vi "Update Command Settings.vi"(8 "error in (no error)":errorcluster, 10 "Command Settings":refnum<class "CommandSetting.lvclass">[](array[class]), 11 "WriteCommand in":refnum<class "WriteCommand.lvclass">) -> (0 "error out":errorcluster, 1 "Updated Count":u32, 2 "Added Count":u32, 3 "WriteCommand out":refnum<class "WriteCommand.lvclass">)   [LabVIEW 2023, in "HAF.lvlib" / "WriteCommand.lvclass"]
doc: "Adds to or updates existing Command Settings on the Command. Returns the number added and updated."
uses:
  WriteCommand.lvclass
  CommandSetting/CommandSetting.lvclass
  WriteCommand.lvclass/WriteCommand.ctl
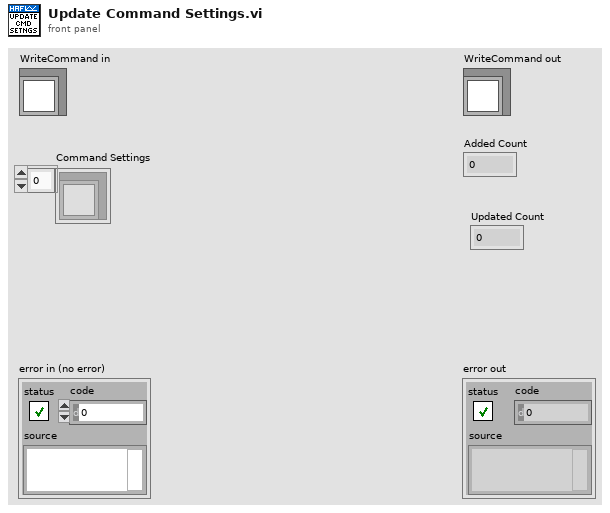
[diagram p1: front panel]
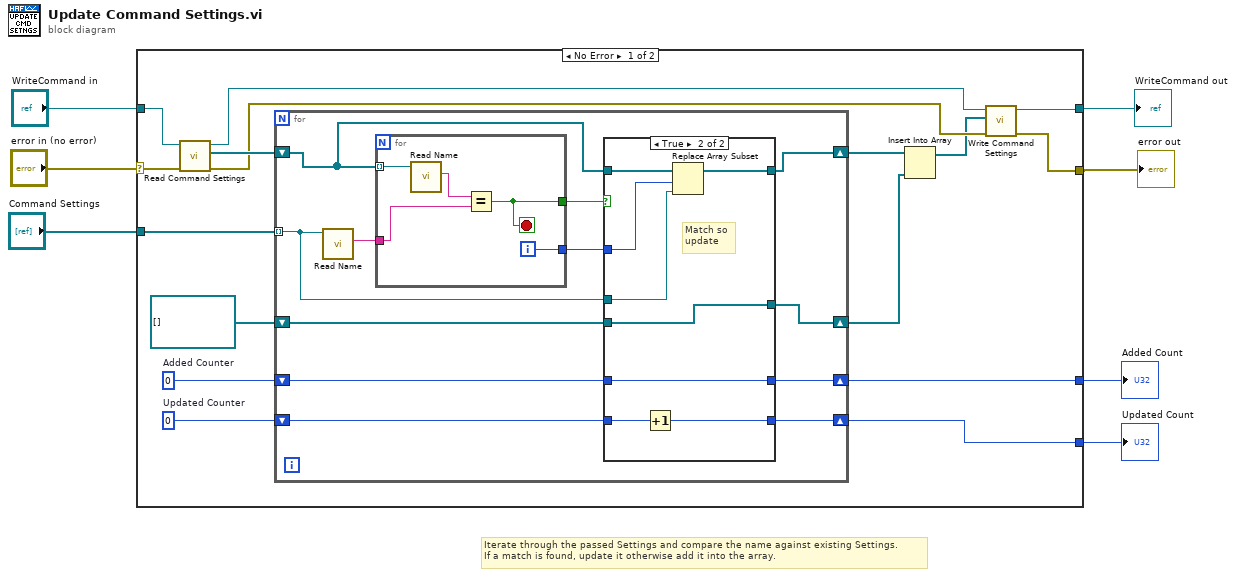
[diagram p0: block diagram]
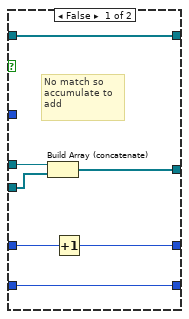
[diagram p2: hidden frame]
diagram:
  # "Iterate through the passed Settings and compare the name against existing Settings.\nIf a match is found, update it otherwise add it into the array."
  n1 = case shown="No Error" "error in (no error)" {
    selector: "error in (no error)" -> [w22 w57]
    tunnel: [w10 w57] -> w3
    tunnel: [w11 w56] -> w4
    tunnel: "WriteCommand in" -> [w23 w56]
    tunnel: "Command Settings" -> [w21 _]
    tunnel: [w9 _] -> w2
    tunnel: [w8 _] -> w1
    frame No Error {
      w18 = u32 0  # Updated Counter
      w19 = u32 0  # Added Counter
      n2 = call-dynamic "Read Command Settings.vi"("error in (no error)"=w22, "WriteCommand in"=w23) -> ("error out"=w14:errorcluster, "Command Settings"=w17:refnum<class "CommandSetting.lvclass">[], "WriteCommand out"=w13:refnum<class "WriteCommand.lvclass">)  [unwired: 7 in]
      n3 = for {
        tunnel: w21 -> [w32] mode=indexing
        shift-right: [w27] -> w15
        shift-left: refnum<class "CommandSetting.lvclass">[] [] -> [w31]
        shift-right: [w26] -> w9
        shift-left: w19 -> [w30]
        shift-right: [w25] -> w8
        shift-left: w18 -> [w29]
        shift-right: [w24] -> w16
        shift-left: w17 -> [w28]
        n4 = call-dynamic "Read Name.vi"("Setting in"=w32) -> ("Name"=w35:string)  [unwired: 8 in, 2 out]
        n5 = for {
          tunnel: w35 -> [w53]
          tunnel: w28 -> [w55] mode=indexing
          tunnel: [w52] -> w34
          tunnel: [w51] -> w33
          i -> [w51]
          stop <- w52 stop-if-true
          n6 = call-dynamic "Read Name.vi"("Setting in"=w55) -> ("Name"=w54:string)  [unwired: 8 in, 2 out]
          n7 = Equal?(x=w54, y=w53) -> (x = y?=w52:bool)
        }
        n8 = case shown="True" w34 {
          tunnel: w33 -> [_ w49]
          tunnel: w32 -> [w41 w48]
          tunnel: w31 -> [w40 w46]
          tunnel: w30 -> [w38 w45]
          tunnel: w29 -> [w36 w44]
          tunnel: w28 -> [w42 w50]
          tunnel: [w42 w47] -> w24
          tunnel: [w39 w46] -> w27
          tunnel: [w37 w45] -> w26
          tunnel: [w36 w43] -> w25
          frame False {
            # "No match so \naccumulate to \nadd"
            n9 = Build Array (concatenate)(w41, w40) -> (w39:refnum<class "CommandSetting.lvclass">[])
            n10 = Increment(x=w38) -> (x+1=w37:u32)
          }
          frame True {
            # "Match so\nupdate"
            n11 = Increment(x=w44) -> (x+1=w43:u32)
            n12 = Replace Array Subset(array=w50, new element=w48, index=w49) -> (w47:refnum<class "CommandSetting.lvclass">[])
          }
        }
      }
      n13 = Insert Into Array(array=w16, new element=w15) -> (w12:refnum<class "CommandSetting.lvclass">[])  [unwired: 1 in]
      n14 = call-dynamic "Write Command Settings.vi"("error in (no error)"=w14, "Command Settings"=w12, "WriteCommand in"=w13) -> ("error out"=w10:errorcluster, "WriteCommand out"=w11:refnum<class "WriteCommand.lvclass">)  [unwired: 7 in]
    }
    frame Error {
    }
  }
  "error out" <- w3
  "WriteCommand out" <- w4
  "Added Count" <- w2
  "Updated Count" <- w1
